vi "Get Active Bool Function.vi"(0 "Bitwise Functions in":refnum<class "Bitwise Functions.lvclass">, 11 "error in (no error)":errorcluster) -> (4 "Bitwise Functions out":refnum<class "Bitwise Functions.lvclass">, 6 "Function":T1, 15 "error out":errorcluster)   [LabVIEW 2016, in "Bitwise Functions.lvclass"]
uses:
  Bitwise Functions.lvclass
  D:/TOOLS/LSL/source code/LSL components/functions/functionsbase/functionbase.lvclass
  Function List.ctl
  functionsbase/functionbase.lvclass
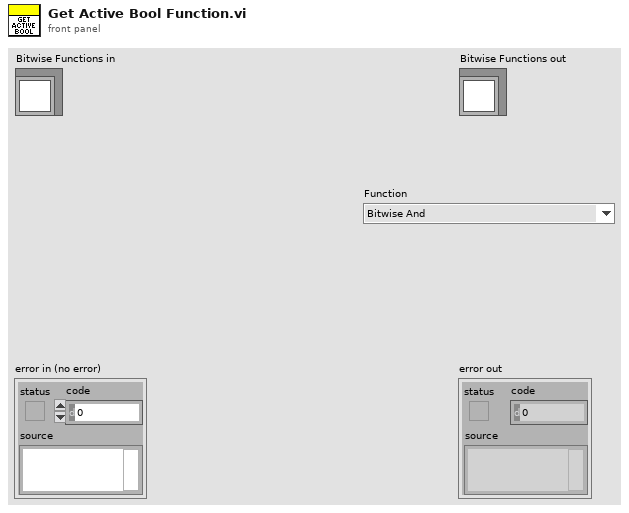
[diagram p1: front panel]
types:
  T1 = typedef "Bitwise Functions.lvclass/Function List.ctl" = enum16{"Bitwise And", "Bitwise Or", "Bitwise ExOR", "One's Compliment", "Shift Left", "Shift Right"}
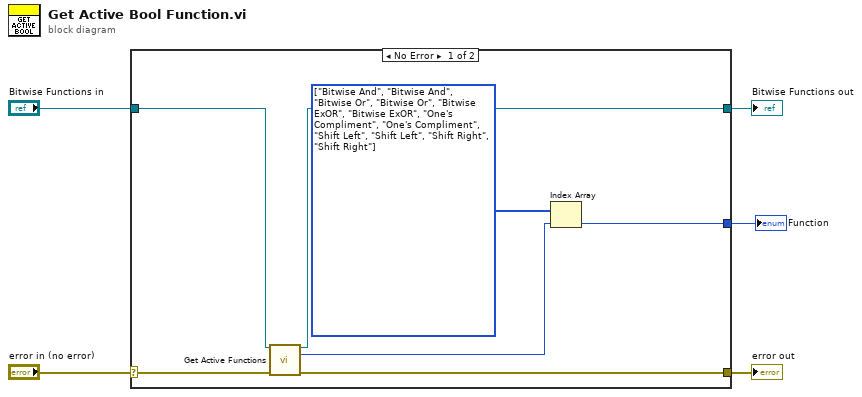
[diagram p0: block diagram]
diagram:
  n1 = case shown="No Error" "error in (no error)" {
    selector: "error in (no error)" -> [w12 w14]
    tunnel: [w11 w14] -> w4
    tunnel: [w9 w13] -> w2
    tunnel: "Bitwise Functions in" -> [w10 w13]
    tunnel: [w6 _] -> w1
    frame No Error {
      w8 = T1[] [enum."Bitwise And", enum."Bitwise And", enum."Bitwise Or", enum."Bitwise Or", enum."Bitwise ExOR", enum."Bitwise ExOR", enum."One's Compliment", enum."One's Compliment", enum."Shift Left", enum."Shift Left", enum."Shift Right", enum."Shift Right"] items=["Bitwise And", "Bitwise Or", "Bitwise ExOR", "One's Compliment", "Shift Left", "Shift Right"]
      n2 = call "Get Active Functions.vi"("functionbase in"=w10, "error in (no error)"=w12) -> ("functionbase out"=w9:refnum<class "Bitwise Functions.lvclass">, "Syntax Index"=w7:i32, "error out"=w11:errorcluster)  [unwired: 11 in]
      n3 = Index Array(array=w8, index=w7) -> (element=w6:T1)
    }
    frame Error {
    }
  }
  "error out" <- w4
  "Bitwise Functions out" <- w2
  "Function" <- w1
